vi "Barrier Destroy.vi"(8 "error in (no error)":errorcluster, 11 "Barrier in":T1) -> (0 "error out":errorcluster, 3 "Barrier out":T1)   [LabVIEW 2016, in "Linux RT IPC.POSIX Threads.lvlib" / "Barrier.lvclass"]
doc: "Calls pthread_barrier_destroy() on the pthread barrier object encapsulated by Barrier.\n\nRefer to online POSIX documentation for more information."
uses:
  Barrier.lvclass
  Controls/reference.ctl
  C:/Git/SourceTree/LinuxRT-IPC/Source/POSIX Threads/Classes/POSIX Thread Object/POSIX Thread Object.lvclass
  POSIX Thread Object/POSIX Thread Object.lvclass/POSIX Thread Object.ctl
  POSIX Thread Object/Private VIs/libpthread path.vi
  POSIX Thread Object/Private VIs/get pthread error.vi
  POSIX Thread Object/POSIX Thread Object.lvclass
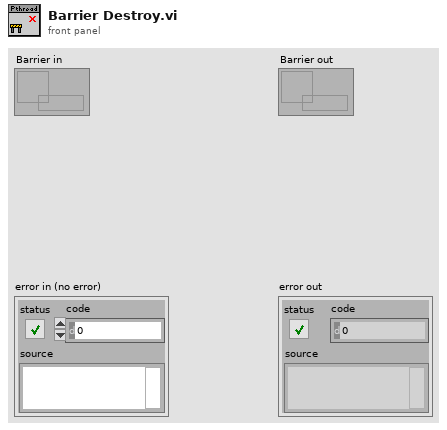
[diagram p1: front panel]
types:
  T1 = typedef "Linux RT IPC.POSIX Threads.lvlib/Barrier.lvclass/reference.ctl" = refnum<data-value>
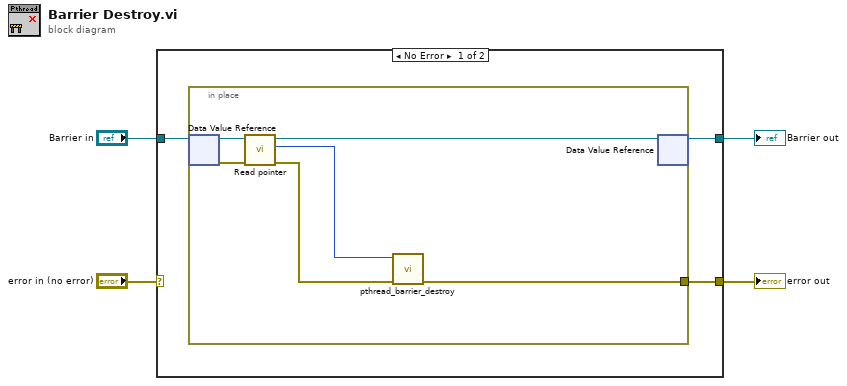
[diagram p0: block diagram]
diagram:
  n1 = case shown="No Error" "error in (no error)" {
    selector: "error in (no error)" -> [_ w15]
    tunnel: [w5 w15] -> w3
    tunnel: "Barrier in" -> [w7 w14]
    tunnel: [w6 w14] -> w1
    frame No Error {
      n2 = in-place {
        in-place-border: [w10] -> w5
        n3 = in-place-dvr #1(w7) -> (w13:refnum<class "Barrier.lvclass">, w11:errorcluster)
        n4 = call "Read pointer.vi"("error in (no error)"=w11, "POSIX Thread Object in"=w13) -> ("error out"=w9:errorcluster, "pointer"=w8:u64, "POSIX Thread Object out"=w12:refnum<class "Barrier.lvclass">)  [unwired: 7 in]
        n5 = call "pthread_barrier_destroy.vi"("error in (no error)"=w9, "barrier ptr in"=w8) -> ("error out"=w10:errorcluster)  [unwired: 8 in, 1 out]
        n6 = in-place-dvr #1(w12) -> (w6:T1)  [unwired: 1 out]
      }
    }
    frame Error {
    }
  }
  "error out" <- w3
  "Barrier out" <- w1
